vi "RT_main_driver_in_RT.vi"() -> ()   [LabVIEW 2016]
doc: "The myRIO Project template acquires acceleration data from the onboard accelerometer and displays the changes of acceleration values in a waveform chart."
uses:
  <vilib>/myRIO/Common/Instrument Driver Framework/myRIO v1.0/UART/vis/myRIO v1.0 Close UART.vi
  <vilib>/Utility/error.llb/Error Cluster From Error Code.vi
  <vilib>/myRIO/Common/Instrument Driver Framework/myRIO v1.0/DIO/vis/myRIO v1.0 Write DIO.vi
  <vilib>/myRIO/Common/Instrument Driver Framework/Utilities/vis/FPGA Ref Manager.vi
  <vilib>/myRIO/Common/Instrument Driver Framework/myRIO v1.0/myRIO v1.0 Reset FPGA.vi
  <vilib>/myRIO/Common/Instrument Driver Framework/myRIO v1.0/IRQ/vis/myRIO v1.0 IRQ Info FGV.vi
  <vilib>/myRIO/Common/Instrument Driver Framework/myRIO v1.0/IRQ/vis/myRIO v1.0 Timer IRQ Info FGV.vi
  <vilib>/myRIO/Common/Instrument Driver Framework/myRIO v1.0/IRQ/vis/myRIO v1.0 ISR Agent.vi
  <vilib>/myRIO/Instrument Drivers/Onboard IO/DIO/DIO.lvlib
  <vilib>/myRIO/Instrument Drivers/Utilities/Utilities.lvlib
panel:
  out "x-y":u32
  in  "Stop Button":bool
  out "error out":errorcluster
  # "Overview: The myRIO Project template acquires acceleration data from the onboard accelerometer and displays the changes of acceleration values in a waveform chart.\nInstructions:\n1. Check the myRIO target IP address in the project and make sure the target IP address is correct. \n2. Run this VI."
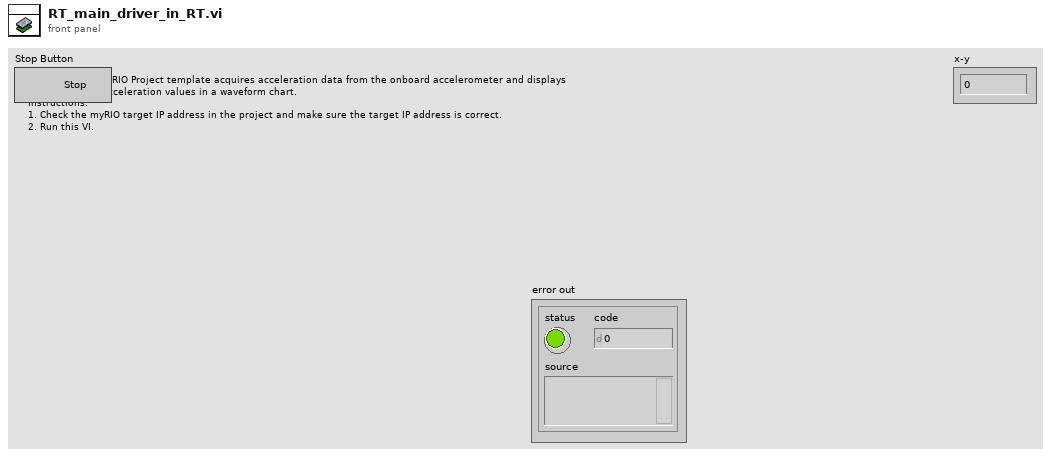
[diagram p1: front panel]
types:
  T1 = typedef "DIO.lvlib/DIO Reference.ctl" = cluster{"myRIO Reference":T2, "DIO Channels List":T6}
  T2 = typedef "myRIO Generic Hardware Reference.ctl" = cluster{"myRIO Model":T3, "myRIO Hardware Reference":T4}
  T3 = typedef "Hardware Version Enum.ctl" = enum16{"Unknown", "myRIO-1900", "myRIO-1950", "roboRIO", "NI ELVIS RIO CM"}
  T4 = typedef "myRIO v1.0 Reference.ctl" = cluster{"Generic FPGA Reference":T5, "Allow multiple opens":bool}
  T5 = typedef "Generic FPGA Reference.ctl" = refnum<k20>
  T6 = typedef "DIO Channels List.ctl" = T7[]
  T7 = typedef "DIO Channels Enum.ctl" = enum16{"Not Connected", "C/DIO0", "C/DIO1", "C/DIO2", "C/DIO3", "C/DIO4", "C/DIO5", "C/DIO6", "C/DIO7", "A/DIO0", "A/DIO1", "A/DIO2", "A/DIO3", "A/DIO4", "A/DIO5", "A/DIO6", "A/DIO7", "A/DIO8", "A/DIO9", "A/DIO10", "A/DIO11", "A/DIO12", "A/DIO13", "A/DIO14", "A/DIO15", "B/DIO0", "B/DIO1", "B/DIO2", "B/DIO3", "B/DIO4", "B/DIO5", "B/DIO6", "B/DIO7", "B/DIO8", "B/DIO9", "B/DIO10", "B/DIO11", "B/DIO12", "B/DIO13", "B/DIO14", "B/DIO15", "LED0", "LED1", "LED2", "LED3", "Button0", "DIO/DIO0", "DIO/DIO1", "DIO/DIO2", "DIO/DIO3", "DIO/DIO4", "DIO/DIO5", "DIO/DIO6", "DIO/DIO7", "DIO/DIO8", "DIO/DIO9", "SPI/CS0", "SPI/CS1", "SPI/CS2", "SPI/CS3", "LED RADIO (Green)", "LED RADIO (Red)", "LED COMM (Green)", "LED COMM (Red)", "LED MODE (Green)", "LED MODE (Red)"}
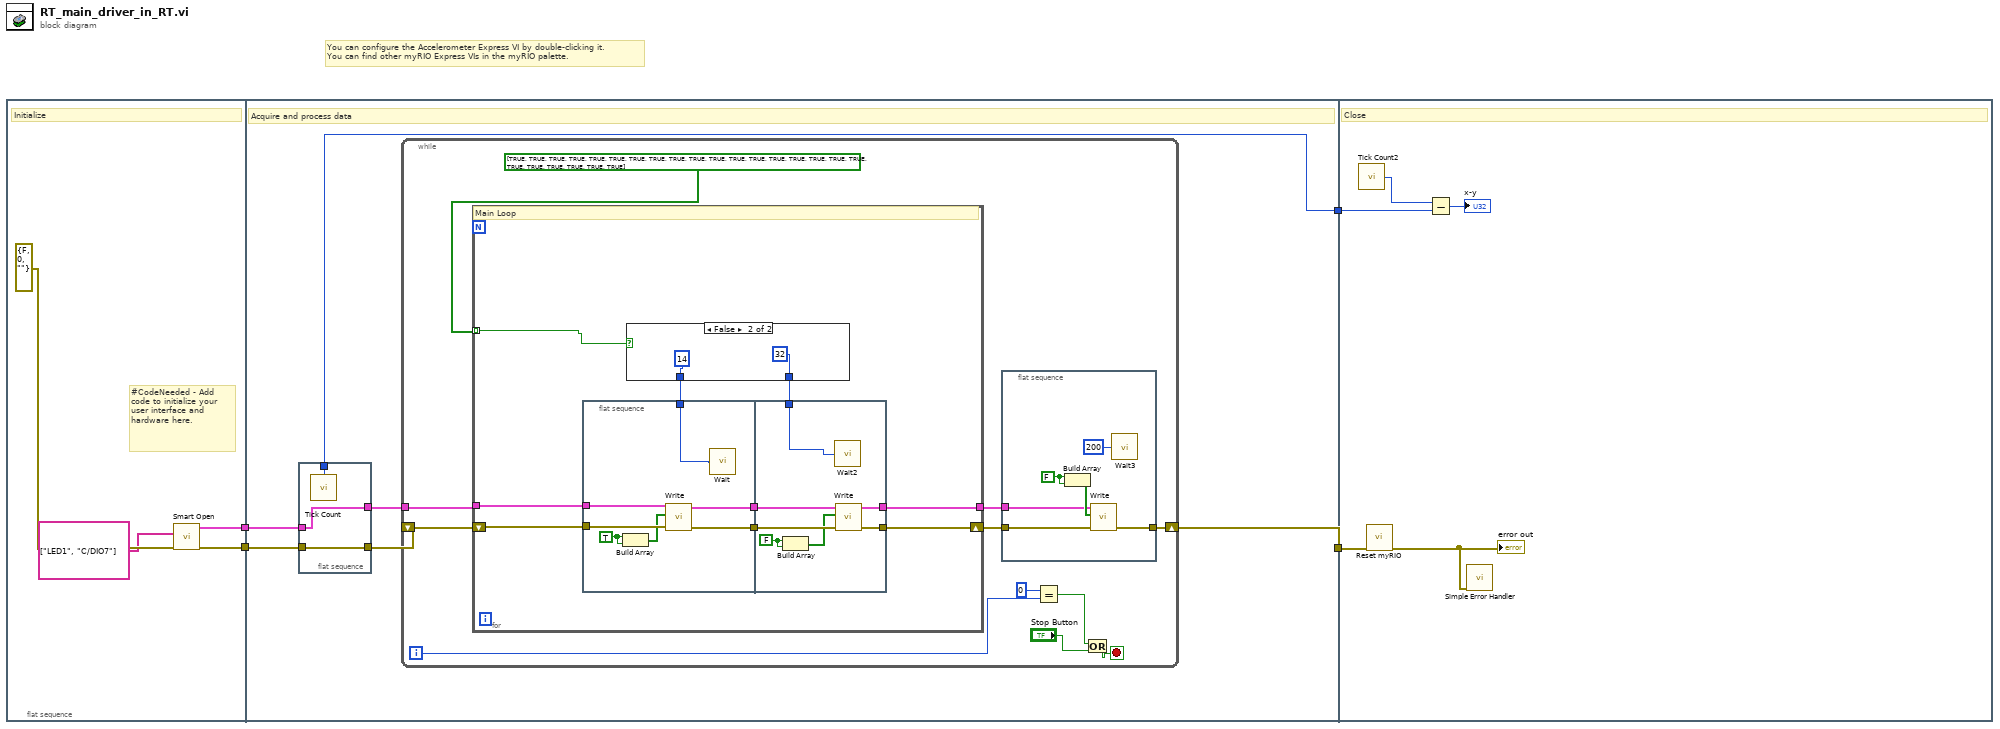
[diagram p0: block diagram]
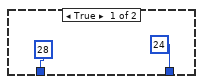
[diagram p2: hidden frame]
diagram:
  # "You can configure the Accelerometer Express VI by double-clicking it.\nYou can find other myRIO Express VIs in the myRIO palette."
  n1 = flat-sequence {
    tunnel: [w7] -> w4
    tunnel: [w5] -> w3
    tunnel: w4 -> [w13]
    tunnel: w3 -> [w11]
    tunnel: [w14] -> w2
    tunnel: [w9] -> w1
    tunnel: w2 -> [w66]
    tunnel: w1 -> [w63]
    frame #0 {
      # "#CodeNeeded - Add code to initialize your user interface and hardware here."
      # "Initialize"
      n2 = call <vilib>:"Smart Open.vi"("error in (no error)"=errorcluster {"status"=FALSE, "code"=0, "source"=""}, "Channel Names"=tag[] ["LED1", "C/DIO7"]) -> ("error out"=w7:errorcluster, "DIO Ref Out"=w5:T1)  [unwired: 8 in]
    }
    frame #1 {
      # "Acquire and process data"
      n3 = flat-sequence {
        tunnel: w13 -> [w17]
        tunnel: [w17] -> w12
        tunnel: w11 -> [w16]
        tunnel: [w16] -> w10
        tunnel: [w15] -> w9
        frame #0 {
          n4 = call "Tick Count"() -> ("Tick Count(uSec)"=w15:u32)
        }
      }
      n5 = while {
        shift-right: [w19] -> w14
        shift-left: w12 -> [w27]
        tunnel: w10 -> [w28]
        i -> [w22]
        stop <- w23 stop-if-true
        n6 = for {
          tunnel: w28 -> [w43]
          tunnel: bool[] [TRUE, TRUE, TRUE, TRUE, TRUE, TRUE, TRUE, TRUE, TRUE, TRUE, TRUE, TRUE, TRUE, TRUE, TRUE, TRUE, TRUE, TRUE, TRUE, TRUE, TRUE, TRUE, TRUE, TRUE] -> [w35] mode=indexing
          tunnel: [w38] -> w18
          shift-right: [w39] -> w20
          shift-left: w27 -> [w42]
          # "Main Loop"
          n7 = flat-sequence {
            tunnel: w43 -> [w54]
            tunnel: w42 -> [w53]
            tunnel: [w52] -> w41
            tunnel: [w50] -> w40
            tunnel: w37 -> [w49]
            tunnel: w41 -> [w61]
            tunnel: w40 -> [w59]
            tunnel: [w58] -> w39
            tunnel: [w57] -> w38
            tunnel: w36 -> [w56]
            frame #0 {
              w48 = TRUE
              n8 = Build Array(w48, w48) -> (w51:bool[])
              n9 = call <vilib>:"Write.vi"("error in (no error)"=w53, "Values"=w51, "DIO Ref In"=w54) -> ("error out"=w52:errorcluster, "DIO Ref Out"=w50:T1)  [unwired: 6 in]
              n10 = call "Wait"("Count(Ticks)"=w49) -> ()  [unwired: 1 out]
            }
            frame #1 {
              w55 = FALSE
              n11 = Build Array(w55, w55) -> (w60:bool[])
              n12 = call "Wait2"("Count(Ticks)"=w56) -> ()  [unwired: 1 out]
              n13 = call <vilib>:"Write.vi"("error in (no error)"=w61, "Values"=w60, "DIO Ref In"=w59) -> ("error out"=w58:errorcluster, "DIO Ref Out"=w57:T1)  [unwired: 6 in]
            }
          }
          n14 = case shown="False" w35 {
            tunnel: [28 14] -> w37
            tunnel: [24 32] -> w36
            frame True {
            }
            frame False {
            }
          }
        }
        n15 = flat-sequence {
          tunnel: w20 -> [w34]
          tunnel: [w33] -> w19
          tunnel: w18 -> [w29]
          frame #0 {
            w32 = FALSE
            n16 = Build Array(w32, w32) -> (w30:bool[])
            n17 = call <vilib>:"Write.vi"("error in (no error)"=w34, "Values"=w30, "DIO Ref In"=w29) -> ("error out"=w33:errorcluster)  [unwired: 6 in, 1 out]
            n18 = call "Wait3"("Count(Ticks)"=u32 200) -> ()  [unwired: 1 out]
          }
        }
        n19 = Equal?(x=0, y=w22) -> (x = y?=w24:bool)
        n20 = Or(x=w24, y="Stop Button") -> (x .or. y?=w23:bool)
      }
    }
    frame #2 {
      # "Close"
      n21 = call "Tick Count2"() -> ("Tick Count(uSec)"=w64:u32)
      n22 = call <vilib>:"Reset myRIO.vi"("error in (no error)"=w66) -> ("error out"=w65:errorcluster)  [unwired: 10 in]
      "error out" <- w65
      n23 = Subtract(x=w64, y=w63) -> (x-y=→"x-y":u32)
      n24 = call <vilib>:"Simple Error Handler.vi"("error in (no error)"=w65) -> ()  [unwired: 4 in, 5 out]
    }
  }
